vi "GenerateFilenames_PCO_IOS.vi"(11 "path":path) -> (0 "TDMS Path":path, 1 "PCO Path":path, 2 "Basler Path":path, 3 "WebCam Path":path, 4 "Analog file name":string="F:\\Data\\130725_14_35_2625", 5 "Basler2 Path":path, 6 "Analog file name (Dev2)":string, 7 "TDMS Path 2":path)   [LabVIEW 2020]
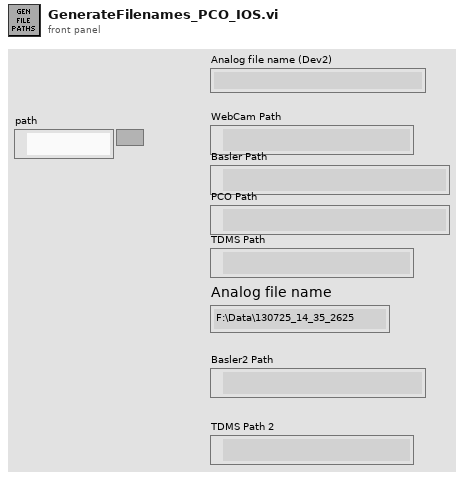
[diagram p1: front panel]
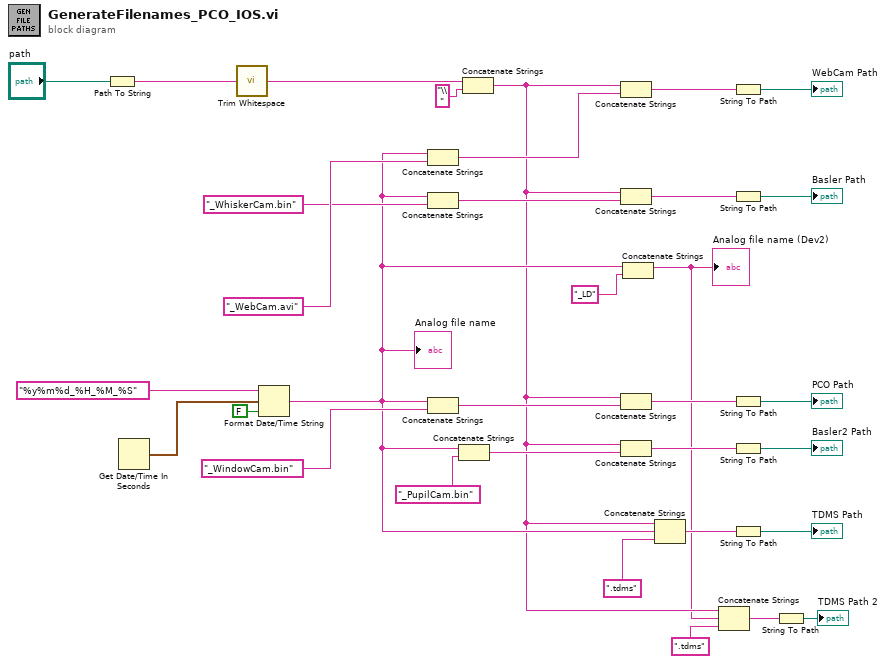
[diagram p0: block diagram]
diagram:
  n1 = Path To String(path="path") -> (string=w15:string)
  n2 = Get Date/Time In Seconds() -> (seconds since 1Jan1904=w32:timestamp)
  n3 = call <vilib>:"Trim Whitespace.vi"("string"=w15) -> ("trimmed string"=w13:string)  [unwired: 1 in]
  n4 = Format Date/Time String(time format string (%c)="%y%m%d_%H_%M_%S", seconds (now)=w32, UTC format=FALSE) -> (date/time string=w7:string)
  "Analog file name" <- w7
  n5 = Concatenate Strings(w7, "_WebCam.avi") -> (w30:string)
  n6 = Concatenate Strings(w7, "_WhiskerCam.bin" ("string")) -> (w24:string)
  n7 = Concatenate Strings(w7, "_WindowCam.bin") -> (w28:string)
  n8 = Concatenate Strings(w7, "_PupilCam.bin" ("string")) -> (w10:string)
  n9 = Concatenate Strings(w13, "\\" ("string")) -> (w2:string)
  n10 = Concatenate Strings(w2, w30) -> (w26:string)
  n11 = Concatenate Strings(w2, w24) -> (w23:string)
  n12 = Concatenate Strings(w2, w28) -> (w27:string)
  n13 = Concatenate Strings(w2, w10) -> (w9:string)
  n14 = Concatenate Strings(w7, "_LD" ("string")) -> (w1:string)
  "Analog file name (Dev2)" <- w1
  n15 = Concatenate Strings(w2, w7, ".tdms" ("string")) -> (w16:string)
  n16 = Concatenate Strings(w2, w1, ".tdms" ("string")) -> (w4:string)
  n17 = String To Path(string=w26) -> (path=→"WebCam Path":path)
  n18 = String To Path(string=w23) -> (path=→"Basler Path":path)
  n19 = String To Path(string=w27) -> (path=→"PCO Path":path)
  n20 = String To Path(string=w9) -> (path=→"Basler2 Path":path)
  n21 = String To Path(string=w16) -> (path=→"TDMS Path":path)
  n22 = String To Path(string=w4) -> (path=→"TDMS Path 2":path)
